vi "niFPGA BW CU Order 1 (32-bit).vi"(0 "filter state in":i32, 1 "reset":bool, 5 "input data":i32, 7 "accumulator in":fxp<+/-,36,32>, 9 "adder in":fxp<+/-,33,33>, 11 "iteration":u8, 12 "In shift":i8=-1, 13 "lowpass?":bool) -> (4 "filter state out":i32, 6 "multiplier":i32, 8 "accumulator out":fxp<+/-,36,32> format="%.14g", 10 "adder out":fxp<+/-,33,33>, 15 "terminate":bool)   [LabVIEW 2017]
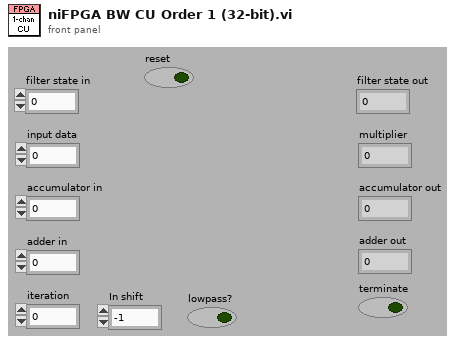
[diagram p1: front panel]
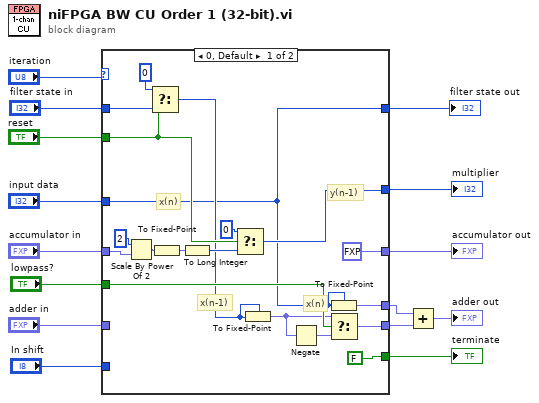
[diagram p0: block diagram]
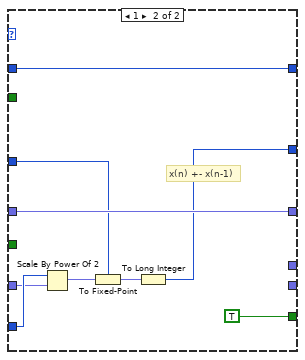
[diagram p2: hidden frame]
diagram:
  n1 = case shown="0, Default" "iteration" {
    tunnel: [w16 w41] -> w11
    tunnel: "input data" -> [w16 w35]
    tunnel: [w25 _] -> w8
    tunnel: "adder in" -> [_ w37]
    tunnel: [w24 w36] -> w10
    tunnel: [w18 _] -> w1
    tunnel: [fxp<+/-,36,32> 0.0 ("Numeric") w42] -> w9
    tunnel: [FALSE TRUE] -> w7
    tunnel: "reset" -> [w29 _]
    tunnel: "accumulator in" -> [w23 w42]
    tunnel: "filter state in" -> [w30 w41]
    tunnel: "In shift" -> [_ w38]
    tunnel: "lowpass?" -> [w27 _]
    frame 0, Default {
      # "x(n)"
      # "x(n-1)"
      # "x(n)"
      # "y(n-1)"
      n2 = Scale By Power Of 2(n=2, x=w23) -> (x*2^n=w20:fxp<+/-,36,32>)
      n3 = Select(t=0 ("filter state in"), s=w29, f=w30) -> (s? t:f=w17:i32)
      n4 = To Fixed-Point(number=w20) -> (fixed-point=w22:fxp<+/-,32,32>)  [unwired: 1 out]
      n5 = To Long Integer(number=w22) -> (32bit integer=w21:i32)
      n6 = Select(t=0, s=w29, f=w21) -> (s? t:f=w24:i32)
      n7 = To Fixed-Point(fixed-point type=w17, number=w17) -> (fixed-point=w19:fxp<+/-,32,32>)
      n8 = Negate(x=w19) -> (-x=w28:fxp<+/-,33,33>)
      n9 = To Fixed-Point(fixed-point type=w16, number=w16) -> (fixed-point=w18:fxp<+/-,32,32>)
      n10 = Select(t=w19, s=w27, f=w28) -> (s? t:f=w25:fxp<+/-,33,33>)
    }
    frame 1 {
      # "x(n) +- x(n-1)"
      n11 = Scale By Power Of 2(n=w38, x=w37) -> (x*2^n=w40:fxp<+/-,33,33>)
      n12 = To Fixed-Point(fixed-point type=w35, number=w40) -> (fixed-point=w39:fxp<+/-,32,32>)
      n13 = To Long Integer(number=w39) -> (32bit integer=w36:i32)
    }
  }
  "multiplier" <- w10
  "terminate" <- w7
  "accumulator out" <- w9
  "filter state out" <- w11
  n14 = Add(x=w1, y=w8) -> (x+y=→"adder out":fxp<+/-,33,33>)
